vi "ex_CM.vi"() -> ()   [LabVIEW 2022 SP3]
doc: "This is the VI which is simple Coffe Machine"
uses:
  #typedef_CM_Operation.ctl
  #typedef_CM_States.ctl
  #typedef_CM_ProgramData.ctl
  #typedef_CM_Kind_Of_Coffe.ctl
  Traffic_Lights/#typedef_TimerAction.ctl
panel:
  in  "Cafe Mocha":bool
  in  "Cafe Latte":bool
  in  "Expresso Machiato":bool
  in  "Expresso":bool
  out "Kind Of Operation":T1
  in  "stop":bool
  # "Wybierz kawe:"
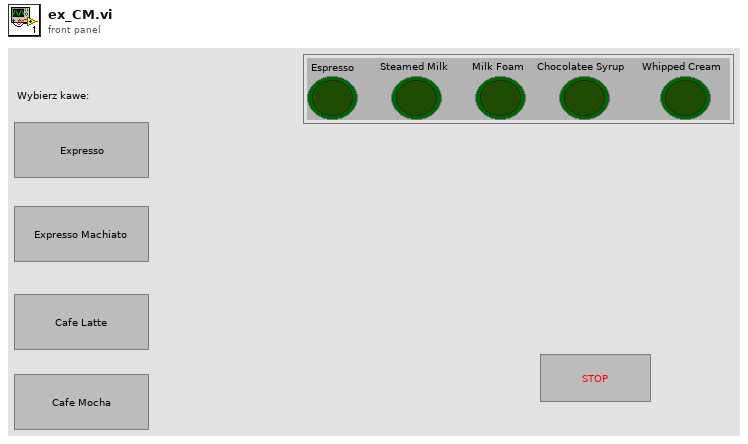
[diagram p1: front panel]
types:
  T1 = typedef "#typedef_CM_Operation.ctl" = cluster{"Espresso":bool, "Steamed Milk":bool, "Milk Foam":bool, "Chocolatee Syrup":bool, "Whipped Cream":bool}
  T2 = typedef "#typedef_CM_States.ctl" = enum16{"Save File", "Whipped Cream", "Chocolate Syrup", "Milk Foam", "Steamed Milk", "Espresso", "Initialize", "Error Handler", "Exit", "Wait For Event"}
  T3 = typedef "#typedef_TimerAction.ctl" = enum16{"Reset", "TimeElapsed"}
  T4 = typedef "#typedef_CM_ProgramData.ctl" = cluster{"Kind Of Operation":T1, "Target Coffe":enum16{"Cafe Mocha", "Cafe Latte", "Expresso Machiato", "Expresso"}, "Kind_Of_Coffe":T5}
  T5 = typedef "#typedef_CM_Kind_Of_Coffe.ctl" = cluster{"Expresso":bool, "Expresso Machiato":bool, "Cafe Latte":bool, "Cafe Mocha":bool}
  T6 = enum16{"Cafe Mocha", "Cafe Latte", "Expresso Machiato", "Expresso"}
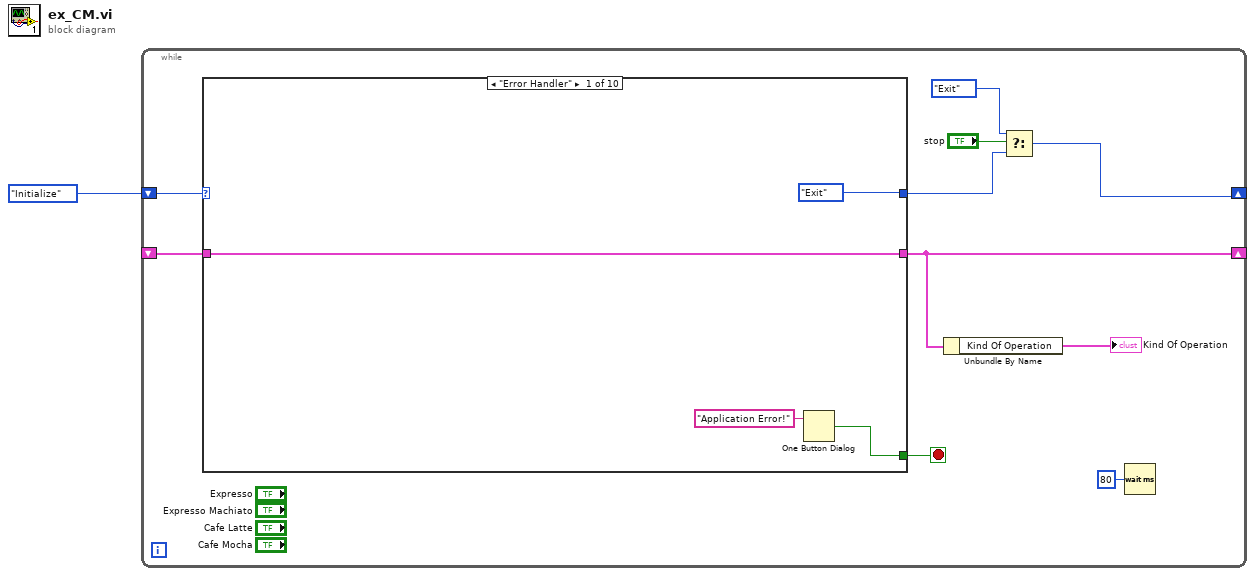
[diagram p0: block diagram]
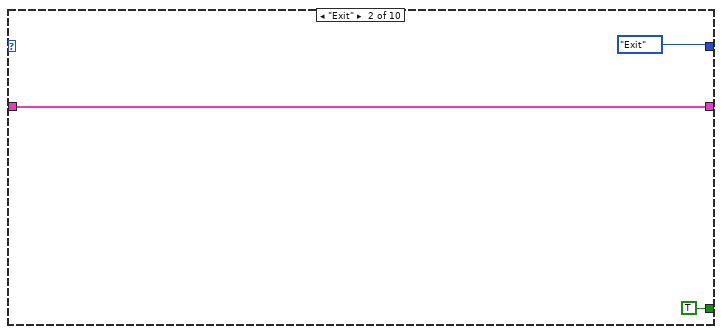
[diagram p2: hidden frame]
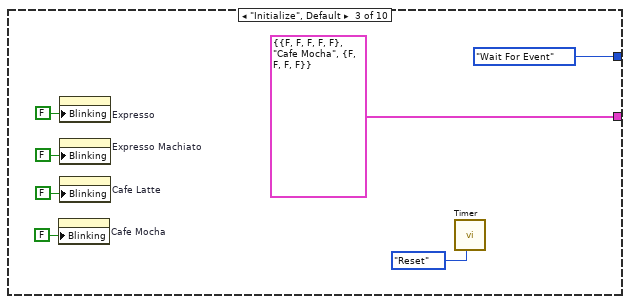
[diagram p3: hidden frame]
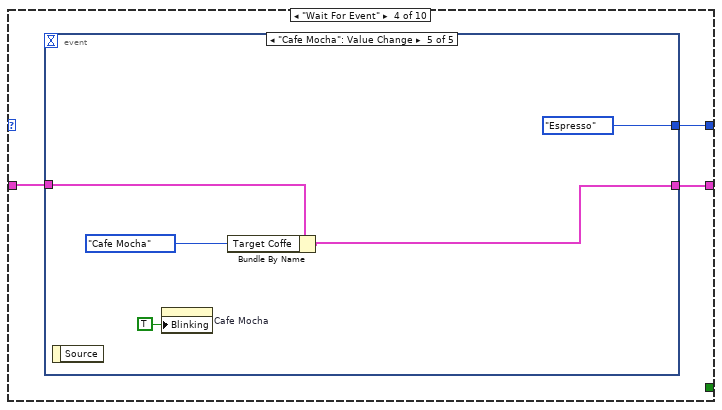
[diagram p4: hidden frame]
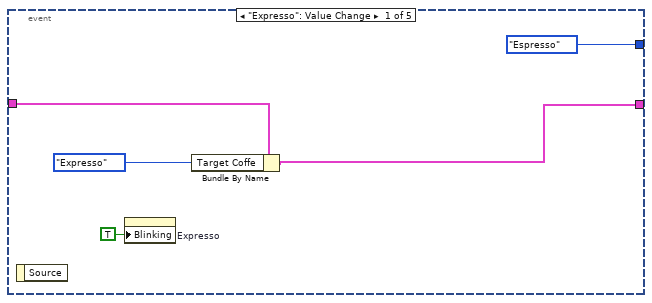
[diagram p5: hidden frame]
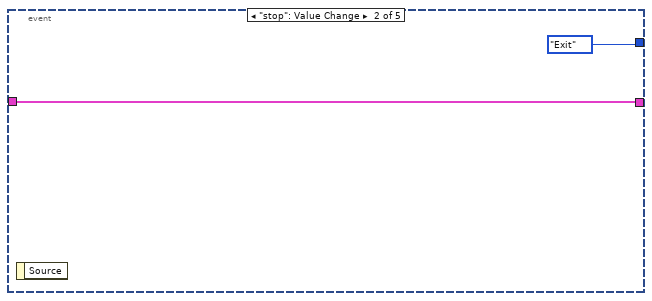
[diagram p6: hidden frame]
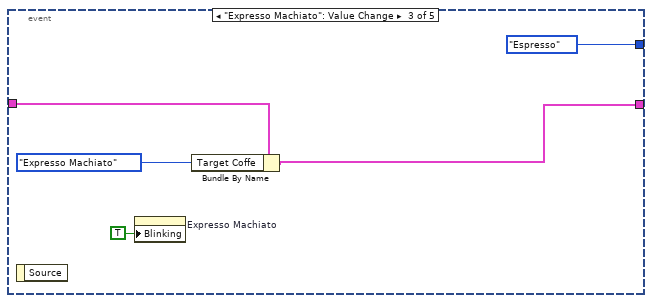
[diagram p7: hidden frame]
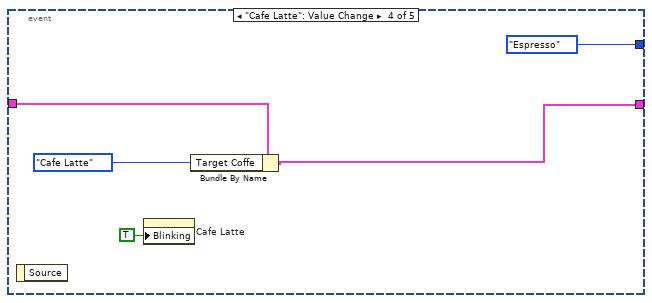
[diagram p8: hidden frame]
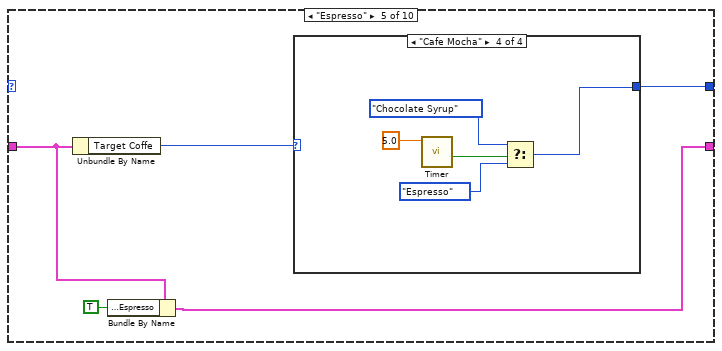
[diagram p9: hidden frame]
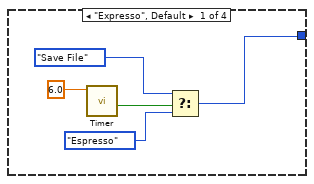
[diagram p10: hidden frame]
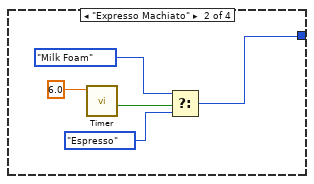
[diagram p11: hidden frame]
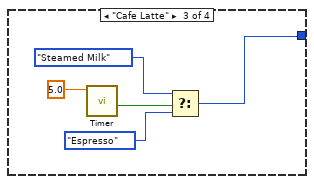
[diagram p12: hidden frame]
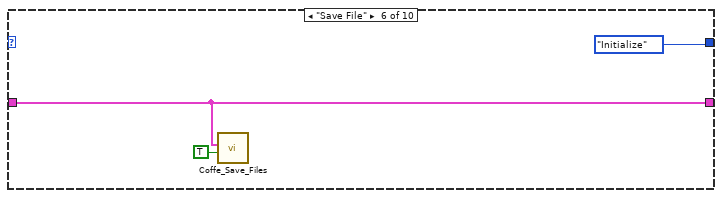
[diagram p13: hidden frame]
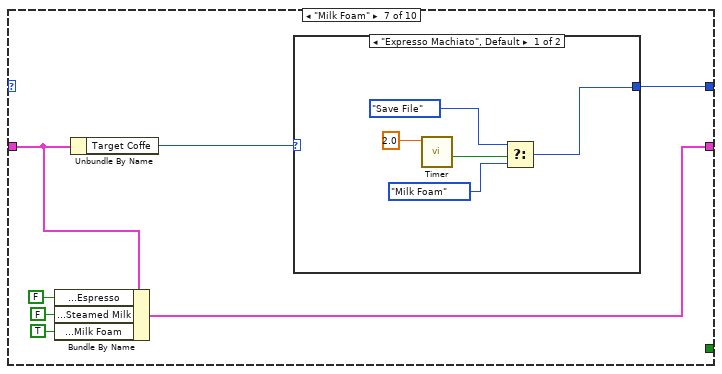
[diagram p14: hidden frame]
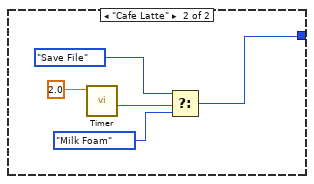
[diagram p15: hidden frame]
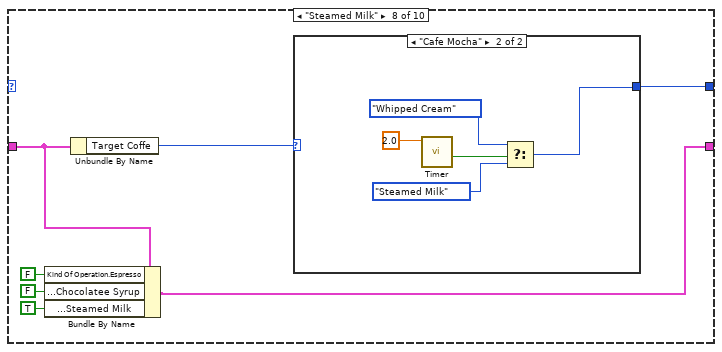
[diagram p16: hidden frame]
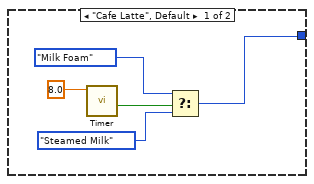
[diagram p17: hidden frame]
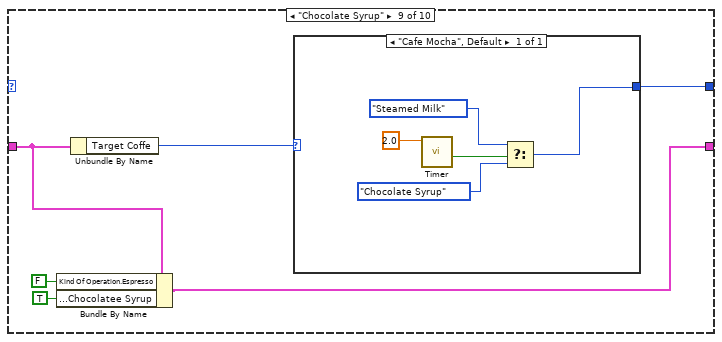
[diagram p18: hidden frame]
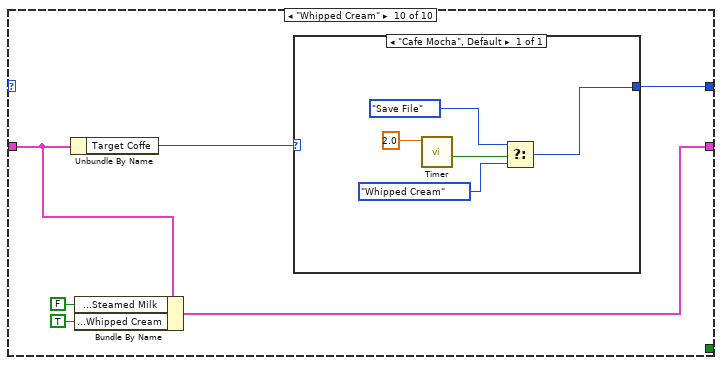
[diagram p19: hidden frame]
diagram:
  n1 = while {
    shift-right: [w6] -> _
    shift-left: #typedef_CM_States."Initialize" ("SM_States") -> [w11]
    shift-right: [w5] -> _
    shift-left: _ -> [w10]
    stop <- w3 stop-if-true
    n2 = case shown="\"Error Handler\"" w11 {
      tunnel: [w13 w16 T4 {"Kind Of Operation"={"Espresso"=FALSE, "Steamed Milk"=FALSE, "Milk Foam"=FALSE, "Chocolatee Syrup"=FALSE, "Whipped Cream"=FALSE}, "Target Coffe"=enum."Cafe Mocha", "Kind_Of_Coffe"={"Expresso"=FALSE, "Expresso Machiato"=FALSE, "Cafe Latte"=FALSE, "Cafe Mocha"=FALSE}} ("Coffe_Machine_ProgramData") w26 w51 w76 w79 w96 w113 w124] -> w5
      tunnel: w10 -> [w13 w16 _ w27 w53 w76 w82 w100 w116 w125]
      tunnel: [#typedef_CM_States."Exit" ("SM_States") #typedef_CM_States."Exit" ("SM_States") #typedef_CM_States."Wait For Event" ("SM_States") w28 w54 #typedef_CM_States."Initialize" ("SM_States") w84 w101 w117 w128] -> w7
      tunnel: [w12 TRUE _ _ _ _ _ _ _ _] -> w3
      frame "Error Handler" {
        n3 = One Button Dialog(message="Application Error!") -> (true=w12:bool)  [unwired: 1 in]
      }
      frame "Exit" {
      }
      frame "Initialize", Default {
        n4 = property on="Cafe Mocha" class="Bool"("Blinking"=FALSE) -> ()  [unwired: 2 in, 2 out]
        n5 = property on="Expresso" class="Bool"("Blinking"=FALSE) -> ()  [unwired: 2 in, 2 out]
        n6 = property on="Expresso Machiato" class="Bool"("Blinking"=FALSE) -> ()  [unwired: 2 in, 2 out]
        n7 = property on="Cafe Latte" class="Bool"("Blinking"=FALSE) -> ()  [unwired: 2 in, 2 out]
        n8 = call "Timer.vi"("Action (Time Elapsed)"=#typedef_TimerAction."Reset") -> ()  [unwired: 8 in, 3 out]
      }
      frame "Wait For Event" {
        n9 = event shown="[4] \"Cafe Mocha\": Value Change" {
          selector: _ -> [_ _ _ _ _]
          dyn-events: _ -> [_ _ _ _ _]
          timeout: _ -> [_ _ _ _ _]
          tunnel: [#typedef_CM_States."Espresso" ("SM_States") #typedef_CM_States."Exit" ("SM_States") #typedef_CM_States."Espresso" ("SM_States") #typedef_CM_States."Espresso" ("SM_States") #typedef_CM_States."Espresso" ("SM_States")] -> w28
          tunnel: w27 -> [w32 w34 w39 w44 w49]
          tunnel: [w30 w34 w37 w42 w47] -> w26
          event "Expresso": Value Change {
            n10 = event-data() -> ()  [unwired: 1 in, 1 out]
            n11 = property on="Expresso" class="Bool"("Blinking"=TRUE) -> ()  [unwired: 2 in, 2 out]
            n12 = Bundle By Name(cluster=w32, "Target Coffe"=T6."Expresso") -> (w30:T4)
          }
          event "stop": Value Change {
            n13 = event-data() -> ()  [unwired: 1 in, 1 out]
          }
          event "Expresso Machiato": Value Change {
            n14 = event-data() -> ()  [unwired: 1 in, 1 out]
            n15 = property on="Expresso Machiato" class="Bool"("Blinking"=TRUE) -> ()  [unwired: 2 in, 2 out]
            n16 = Bundle By Name(cluster=w39, "Target Coffe"=T6."Expresso Machiato") -> (w37:T4)
          }
          event "Cafe Latte": Value Change {
            n17 = event-data() -> ()  [unwired: 1 in, 1 out]
            n18 = property on="Cafe Latte" class="Bool"("Blinking"=TRUE) -> ()  [unwired: 2 in, 2 out]
            n19 = Bundle By Name(cluster=w44, "Target Coffe"=T6."Cafe Latte") -> (w42:T4)
          }
          event "Cafe Mocha": Value Change {
            n20 = event-data() -> ()  [unwired: 1 in, 1 out]
            n21 = property on="Cafe Mocha" class="Bool"("Blinking"=TRUE) -> ()  [unwired: 2 in, 2 out]
            n22 = Bundle By Name(cluster=w49, "Target Coffe"=T6."Cafe Mocha") -> (w47:T4)
          }
        }
      }
      frame "Espresso" {
        n23 = Unbundle By Name(w53) -> ("Target Coffe"=w55:T6)
        n24 = Bundle By Name(cluster=w53, "Kind Of Operation.Espresso"=TRUE) -> (w51:T4)
        n25 = case shown="\"Cafe Mocha\"" w55 {
          tunnel: [w56 w61 w66 w71] -> w54
          frame "Expresso", Default {
            n26 = call "Timer.vi"("Time To Elapse"=6.0) -> ("Time Elapsed?"=w59:bool)  [unwired: 8 in, 2 out]
            n27 = Select(t=#typedef_CM_States."Save File" ("SM_States"), s=w59, f=#typedef_CM_States."Espresso") -> (s? t:f=w56:T2)
          }
          frame "Expresso Machiato" {
            n28 = call "Timer.vi"("Time To Elapse"=6.0) -> ("Time Elapsed?"=w64:bool)  [unwired: 8 in, 2 out]
            n29 = Select(t=#typedef_CM_States."Milk Foam" ("SM_States"), s=w64, f=#typedef_CM_States."Espresso") -> (s? t:f=w61:T2)
          }
          frame "Cafe Latte" {
            n30 = call "Timer.vi"("Time To Elapse"=5.0) -> ("Time Elapsed?"=w69:bool)  [unwired: 8 in, 2 out]
            n31 = Select(t=#typedef_CM_States."Steamed Milk" ("SM_States"), s=w69, f=#typedef_CM_States."Espresso") -> (s? t:f=w66:T2)
          }
          frame "Cafe Mocha" {
            n32 = call "Timer.vi"("Time To Elapse"=5.0) -> ("Time Elapsed?"=w74:bool)  [unwired: 8 in, 2 out]
            n33 = Select(t=#typedef_CM_States."Chocolate Syrup" ("SM_States"), s=w74, f=#typedef_CM_States."Espresso") -> (s? t:f=w71:T2)
          }
        }
      }
      frame "Save File" {
        n34 = call "Coffe_Save_Files.vi"("Is Coffe Done?"=TRUE, "Coffe_Machine_ProgramData"=w76) -> ()  [unwired: 9 in, 1 out]
      }
      frame "Milk Foam" {
        n35 = Bundle By Name(cluster=w82, "Kind Of Operation.Espresso"=FALSE, "Kind Of Operation.Steamed Milk"=FALSE, "Kind Of Operation.Milk Foam"=TRUE) -> (w79:T4)
        n36 = Unbundle By Name(w82) -> ("Target Coffe"=w85:T6)
        n37 = case shown="\"Expresso Machiato\", Default" w85 {
          tunnel: [w86 w91] -> w84
          frame "Expresso Machiato", Default {
            n38 = call "Timer.vi"("Time To Elapse"=2.0) -> ("Time Elapsed?"=w89:bool)  [unwired: 8 in, 2 out]
            n39 = Select(t=#typedef_CM_States."Save File" ("SM_States"), s=w89, f=#typedef_CM_States."Milk Foam") -> (s? t:f=w86:T2)
          }
          frame "Cafe Latte" {
            n40 = call "Timer.vi"("Time To Elapse"=2.0) -> ("Time Elapsed?"=w94:bool)  [unwired: 8 in, 2 out]
            n41 = Select(t=#typedef_CM_States."Save File" ("SM_States"), s=w94, f=#typedef_CM_States."Milk Foam") -> (s? t:f=w91:T2)
          }
        }
      }
      frame "Steamed Milk" {
        n42 = Bundle By Name(cluster=w100, "Kind Of Operation.Espresso"=FALSE, "Kind Of Operation.Chocolatee Syrup"=FALSE, "Kind Of Operation.Steamed Milk"=TRUE ("Kind Of Operation.Milk Foam")) -> (w96:T4)
        n43 = Unbundle By Name(w100) -> ("Target Coffe"=w102:T6)
        n44 = case shown="\"Cafe Mocha\"" w102 {
          tunnel: [w103 w108] -> w101
          frame "Cafe Latte", Default {
            n45 = call "Timer.vi"("Time To Elapse"=8.0) -> ("Time Elapsed?"=w106:bool)  [unwired: 8 in, 2 out]
            n46 = Select(t=#typedef_CM_States."Milk Foam" ("SM_States"), s=w106, f=#typedef_CM_States."Steamed Milk") -> (s? t:f=w103:T2)
          }
          frame "Cafe Mocha" {
            n47 = call "Timer.vi"("Time To Elapse"=2.0) -> ("Time Elapsed?"=w111:bool)  [unwired: 8 in, 2 out]
            n48 = Select(t=#typedef_CM_States."Whipped Cream" ("SM_States"), s=w111, f=#typedef_CM_States."Steamed Milk") -> (s? t:f=w108:T2)
          }
        }
      }
      frame "Chocolate Syrup" {
        n49 = Bundle By Name(cluster=w116, "Kind Of Operation.Espresso"=FALSE, "Kind Of Operation.Chocolatee Syrup"=TRUE) -> (w113:T4)
        n50 = Unbundle By Name(w116) -> ("Target Coffe"=w118:T6)
        n51 = case shown="\"Cafe Mocha\", Default" w118 {
          tunnel: [w119] -> w117
          frame "Cafe Mocha", Default {
            n52 = call "Timer.vi"("Time To Elapse"=2.0) -> ("Time Elapsed?"=w122:bool)  [unwired: 8 in, 2 out]
            n53 = Select(t=#typedef_CM_States."Steamed Milk" ("SM_States"), s=w122, f=#typedef_CM_States."Chocolate Syrup") -> (s? t:f=w119:T2)
          }
        }
      }
      frame "Whipped Cream" {
        n54 = Unbundle By Name(w125) -> ("Target Coffe"=w129:T6)
        n55 = Bundle By Name(cluster=w125, "Kind Of Operation.Steamed Milk"=FALSE, "Kind Of Operation.Whipped Cream"=TRUE) -> (w124:T4)
        n56 = case shown="\"Cafe Mocha\", Default" w129 {
          tunnel: [w130] -> w128
          frame "Cafe Mocha", Default {
            n57 = call "Timer.vi"("Time To Elapse"=2.0) -> ("Time Elapsed?"=w133:bool)  [unwired: 8 in, 2 out]
            n58 = Select(t=#typedef_CM_States."Save File" ("SM_States"), s=w133, f=#typedef_CM_States."Whipped Cream") -> (s? t:f=w130:T2)
          }
        }
      }
    }
    n59 = Unbundle By Name(w5) -> ("Kind Of Operation"=→"Kind Of Operation":T1)
    n60 = Select(t=#typedef_CM_States."Exit" ("SM_States"), s="stop", f=w7) -> (s? t:f=w6:T2)
    n61 = Wait (ms)(milliseconds to wait=u32 80) -> ()  [unwired: 1 out]
  }
